vi "brc_daq_set_parameters.vi"(0 "sample_rate":dbl, 1 "coupling_mode":i32, 2 "current_mA":dbl, 5 "error in (no error)":errorcluster, 6 "mHandle":i32) -> (19 "error out":errorcluster)   [LabVIEW 2015, in "BRC-DAQ x64.lvlib"]
uses:
  BRC-DAQ x64.lvlib
  DLL/brc_daq_sdk.dll
panel:
  out "return_value":i32
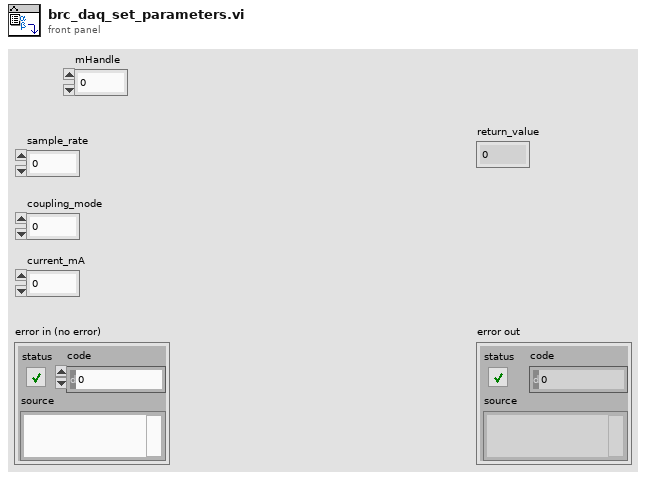
[diagram p1: front panel]
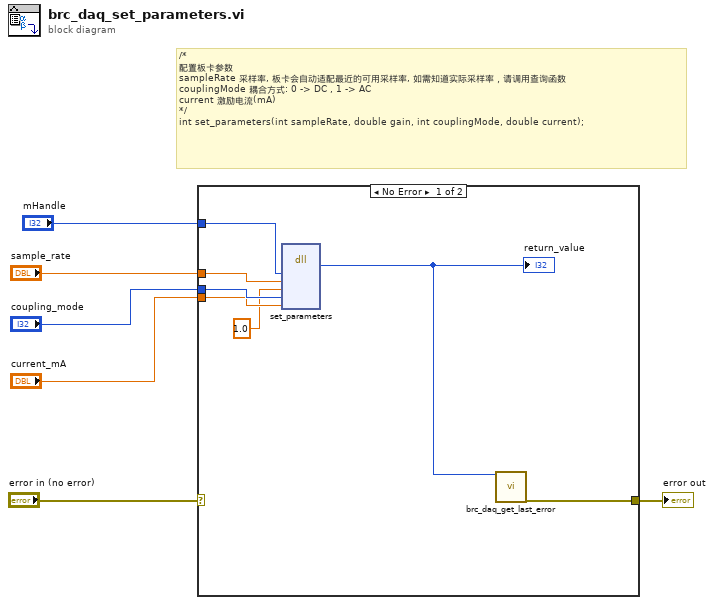
[diagram p0: block diagram]
diagram:
  # "/*\n配置板卡参数\nsampleRate 采样率, 板卡会自动适配最近的可用采样率, 如需知道实际采样率，请调用查询函数\ncouplingMode 耦合方式: 0 -> DC , 1 -> AC\ncurrent 激励电流(mA)\n*/\nint set_parameters(int sampleRate, double gain, int couplingMode, double current);"
  n1 = case shown="No Error" "error in (no error)" {
    selector: "error in (no error)" -> [_ w14]
    tunnel: "sample_rate" -> [w13 _]
    tunnel: "coupling_mode" -> [w12 _]
    tunnel: "current_mA" -> [w11 _]
    tunnel: [w9 w14] -> w3
    tunnel: "mHandle" -> [w7 _]
    frame No Error {
      n2 = dll-call lib="E:/01 BRC project/04BRC-daq/04 Drive/BRC-DAQ/DAQ-x64/DLL/brc_daq_sdk.dll" fn="set_parameters"("mHandle"=w7, "sampleRate"=w13, "gain"=1.0, "couplingMode"=w12, "current"=w11) -> ("return type"=w10:i32)  [unwired: 8 in, 2 out]
      "return_value" <- w10
      n3 = call "brc_daq_get_last_error.vi"("return_value"=w10) -> ("error out"=w9:errorcluster)  [unwired: 18 in]
    }
    frame Error {
    }
  }
  "error out" <- w3
